vi "DisableOutput.vi"(8 "error in (no error)":errorcluster, 11 "FGEN Resource Name":refnum<k15>) -> (0 "error out":errorcluster, 3 "Instrument Handle Out":refnum<k15>)   [LabVIEW 2020]
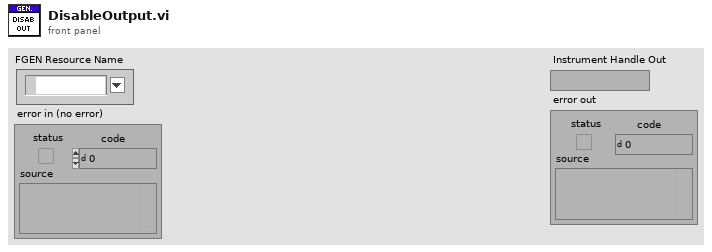
[diagram p1: front panel]
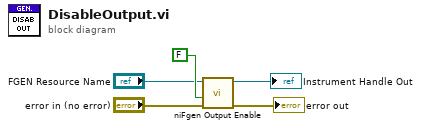
[diagram p0: block diagram]
diagram:
  n1 = call <instrlib>:"niFgen Output Enable.vi"("error in (no error)"="error in (no error)", "Output Enable (default: True)"=FALSE ("output enable"), "Instrument Handle"="FGEN Resource Name") -> ("error out"=→"error out":errorcluster, "Instrument Handle Out"=→"Instrument Handle Out":refnum<k15>)  [unwired: 7 in]
